vi "Write Legend Disable.vi"(5 "Legend Disable":bool, 9 "WaveformChart in":refnum<class "WaveformGraph.lvclass">) -> (3 "WaveformChart out":refnum<class "WaveformGraph.lvclass">)   [LabVIEW 2014, in "WaveformGraph.lvclass"]
uses:
  WaveformGraph.lvclass
  WaveformGraph.lvclass/WaveformGraph.ctl
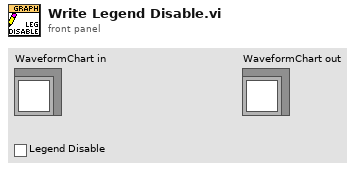
[diagram p1: front panel]
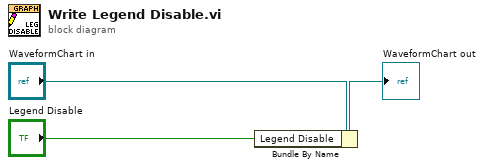
[diagram p0: block diagram]
diagram:
  n1 = Bundle By Name(cluster="WaveformChart in", "Legend Disable"="Legend Disable") -> (→"WaveformChart out":refnum<class "WaveformGraph.lvclass">)
